vi "DIO Block Read Bank.vi"(8 "DI.DMA_ENA":T1, 9 "DATA IN":fxp<+,20,20>, 10 "DI.DMA_CNTR":u16, 11 "DMA FIFO In":refnum<k21>="DI") -> (0 "DI.DMA_IDL":bool)   [LabVIEW 2021]
uses:
  <vilib>/rvi/DataTransferAndStorage/Container/XNode/niFpgaContainer.xnode
  <vilib>/rvi/FIFO/Fifo_Resource/niFpgaFifoEmulationRefIn.vi
  Utilities/Start Boolean.ctl
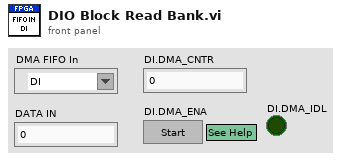
[diagram p1: front panel]
types:
  T1 = typedef "Start Boolean.ctl" = bool
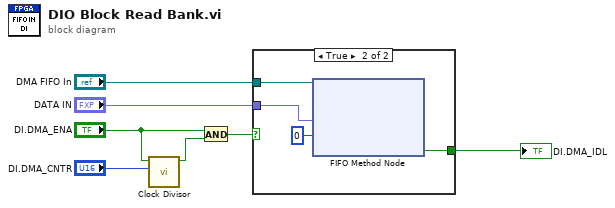
[diagram p0: block diagram]
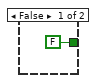
[diagram p2: hidden frame]
diagram:
  n1 = call "Clock Divisor.vi"("Count Number"="DI.DMA_CNTR", "Trigger"="DI.DMA_ENA") -> ("Finished"=w5:bool)  [unwired: 9 in]
  n2 = And(x="DI.DMA_ENA", y=w5) -> (x .and. y?=w4:T1)
  n3 = case shown="True" w4 {
    tunnel: "DMA FIFO In" -> [_ w12]
    tunnel: "DATA IN" -> [_ w11]
    tunnel: [FALSE ("Timed Out?") w9] -> w1
    frame False {
    }
    frame True {
      n4 = xnode ("FIFO Method Node")("Element"=w11, "Timeout"=0, "FIFO In"=w12) -> ("Timed Out?"=w9:bool)  [unwired: 1 out]
    }
  }
  "DI.DMA_IDL" <- w1
